vi "MotionMacro#CMDExecute.vi"(3 "ProgramRef":refnum<vi>, 4 "Command":string[](array[string]), 5 "ThreadsQueue":refnum<queue>[](array[refnum]), 6 "ThreadNo.":u32, 7 "ThreadModReceive":refnum<queue>[](array[refnum]), 8 "StackIn":cluster{"Program":i32, "Prog Index":i32}[](array[cluster]), 9 "ThreadInfoIn":T1) -> (0 "StackOut":cluster{"Program":i32, "Prog Index":i32}[](array[cluster]), 1 "ThreadInfoOut":T1, 2 "ErrorCode":string)   [LabVIEW 2020]
uses:
  MainFrame/Global.vi
panel:
  out "Macro":string[][](array[string])
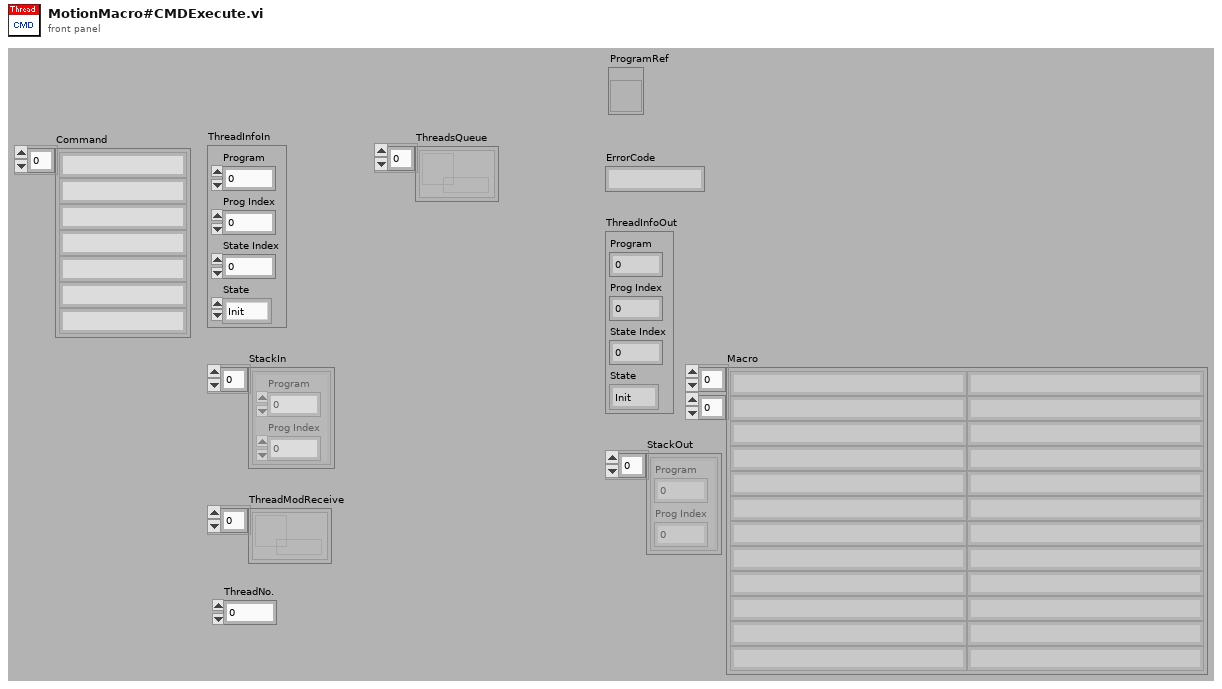
[diagram p1: front panel]
types:
  T1 = cluster{"Program":i32, "Prog Index":i32, "State Index":i32, "State":enum16{"Init", "Idle", "Auto Start", "Auto Running", "Step Start", "Step Running", "Suspend", "Restart", "Stop", "Reset"}}
  T2 = cluster{"指令":string, "代碼":string, "參數長度":i32, "乘數":dbl, "加數":dbl}[]
  T3 = enum16{"Get", "Init", "Set", "Delete", "GetElement", "Inc", "Dec", "ReName", "Copy"}
  T4 = enum16{"Init", "Idle", "Auto Start", "Auto Running", "Step Start", "Step Running", "Suspend", "Restart", "Stop", "Reset"}
  T5 = enum16{"Get", "UpdatePointS", "Init", "UpdateIndex", "GetCurrent&Index+1", "GetWithIndex", "ChkLast"}
  T6 = cluster{"指令":string, "代碼":string, "參數長度":i32, "乘數":dbl, "加數":dbl}[][]
  T7 = cluster{"指令":string, "代碼":string, "參數長度":i32, "乘數":dbl, "加數":dbl}
  T8 = cluster{cluster{"X":sgl, "Y":sgl, "Z":sgl, "U":sgl, "V":sgl, "W":sgl, "H":sgl}[]}
  T9 = cluster{"X":sgl, "Y":sgl, "Z":sgl, "U":sgl, "V":sgl, "W":sgl, "H":sgl}[]
  T10 = cluster{"X":sgl, "Y":sgl, "Z":sgl, "U":sgl, "V":sgl, "W":sgl, "H":sgl}
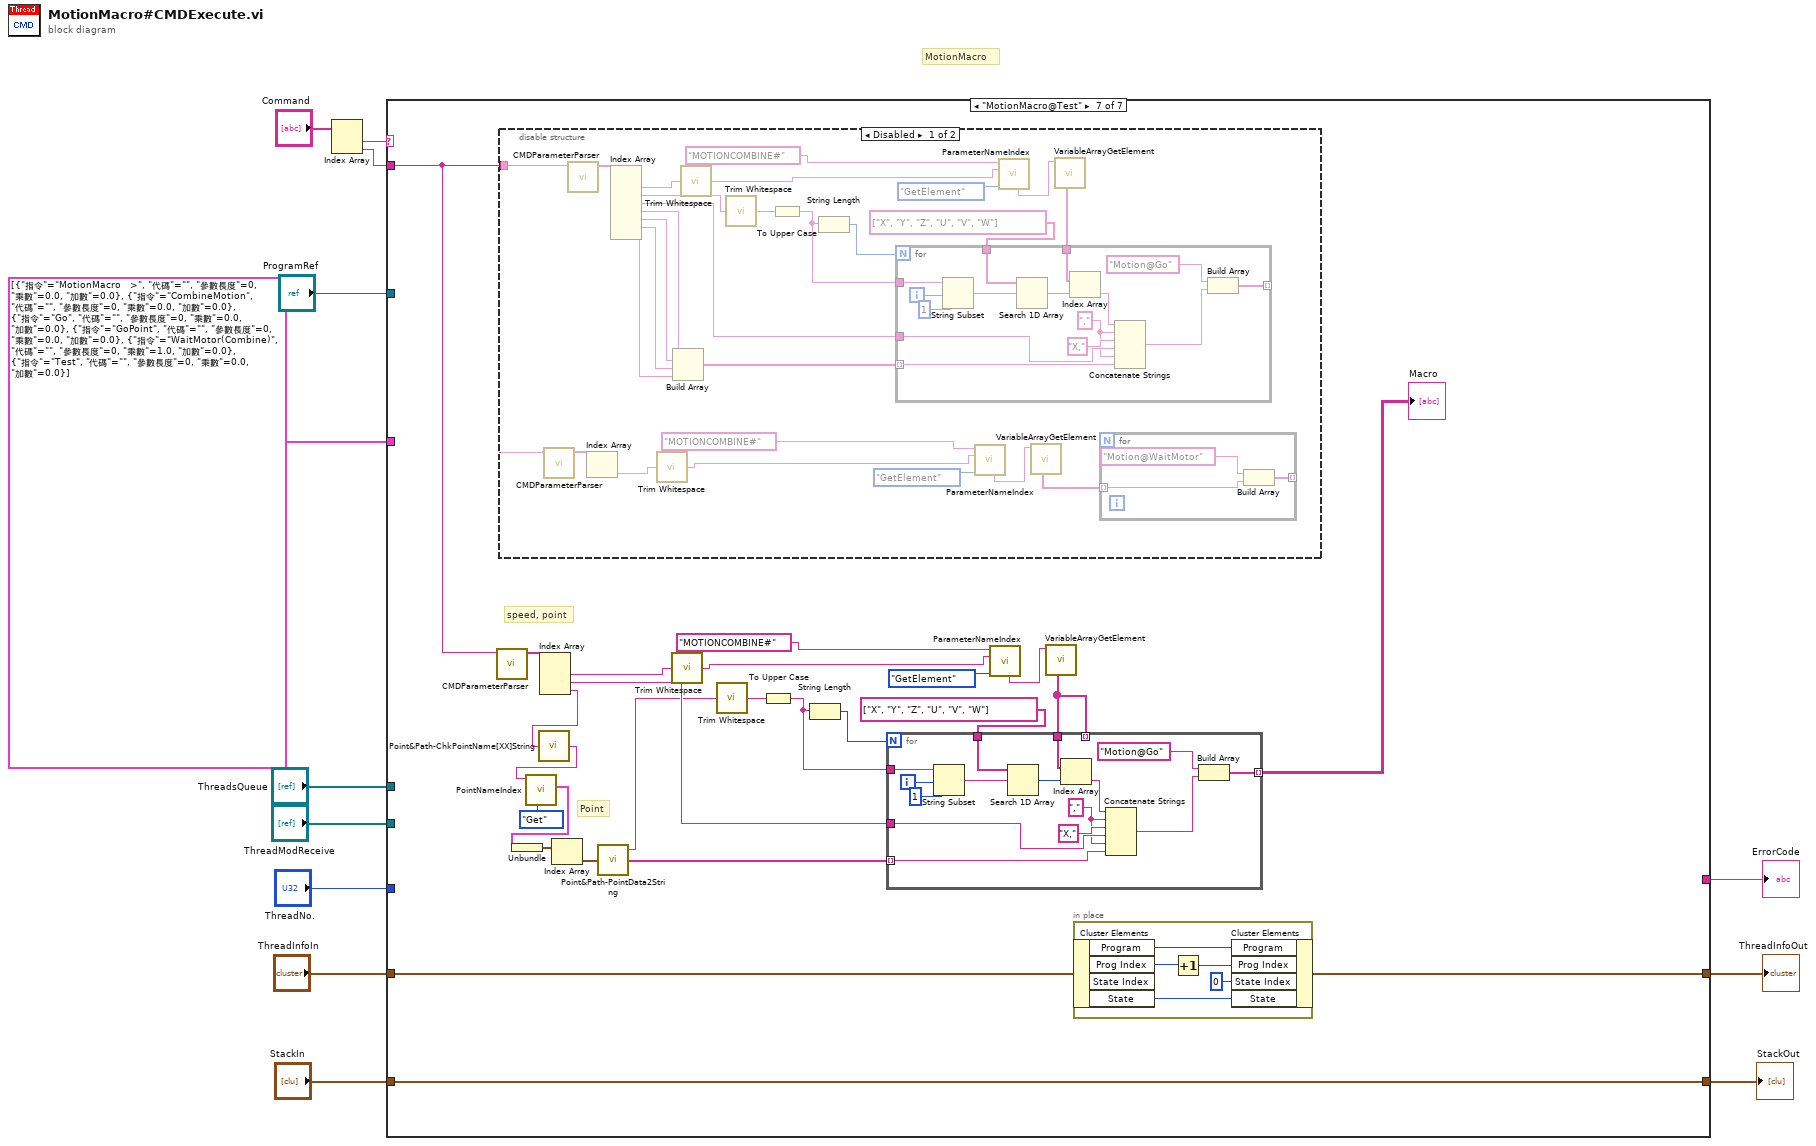
[diagram p0: block diagram]
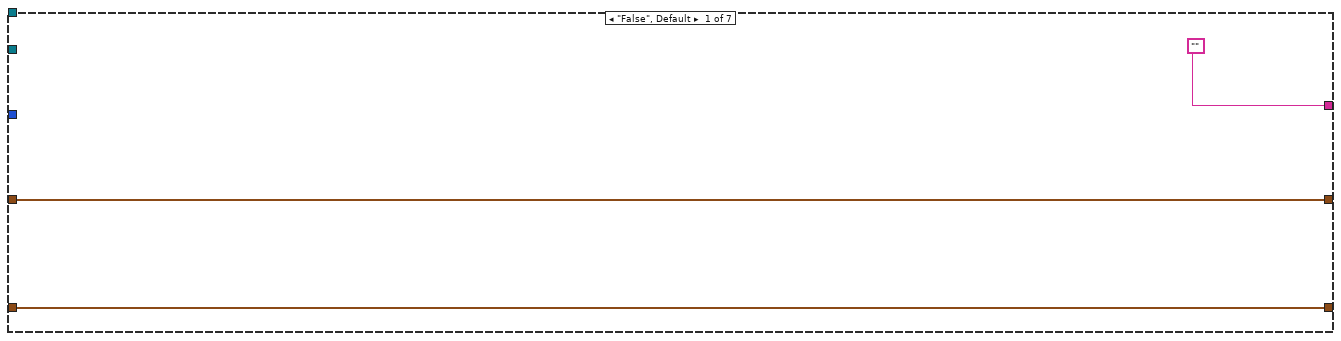
[diagram p2: hidden frame]
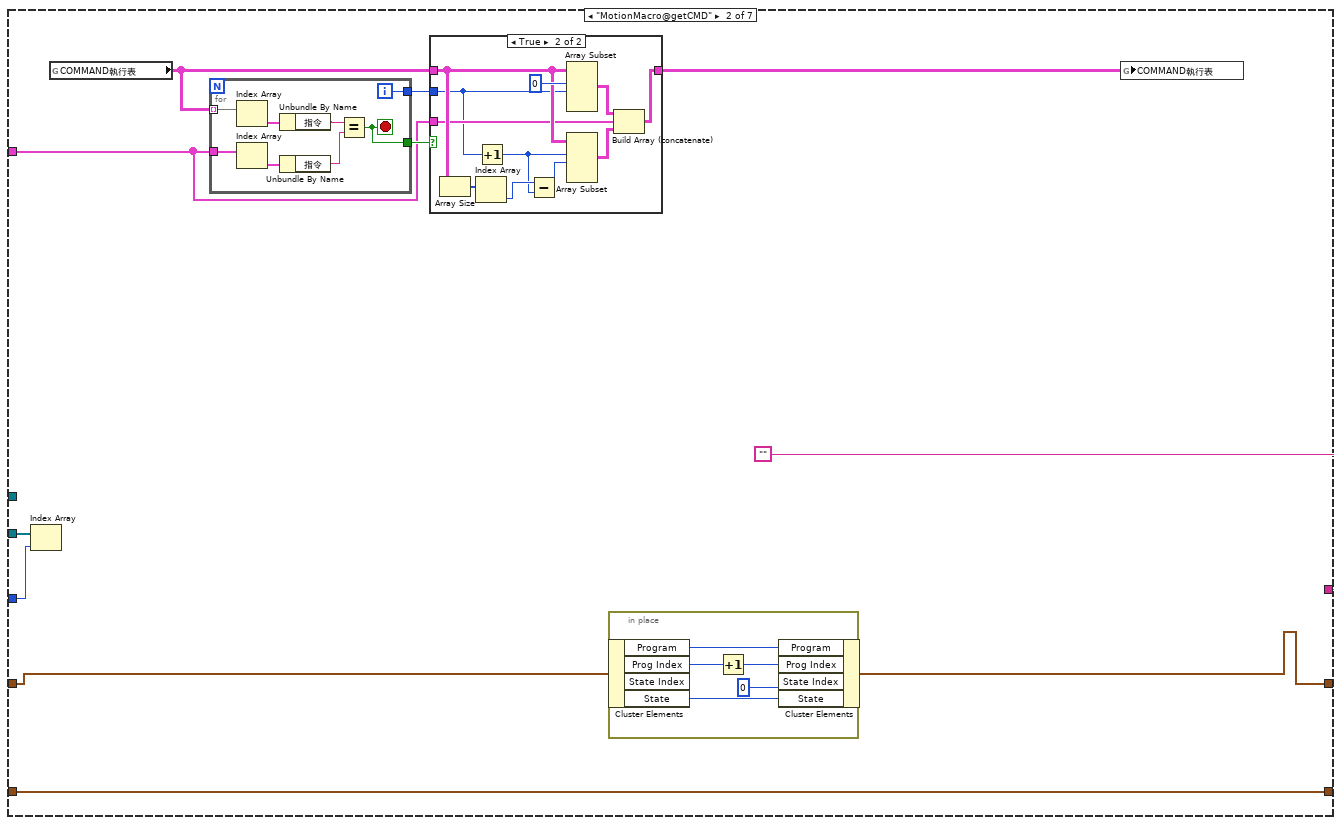
[diagram p3: hidden frame]
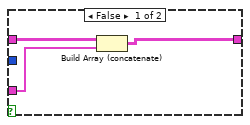
[diagram p4: hidden frame]
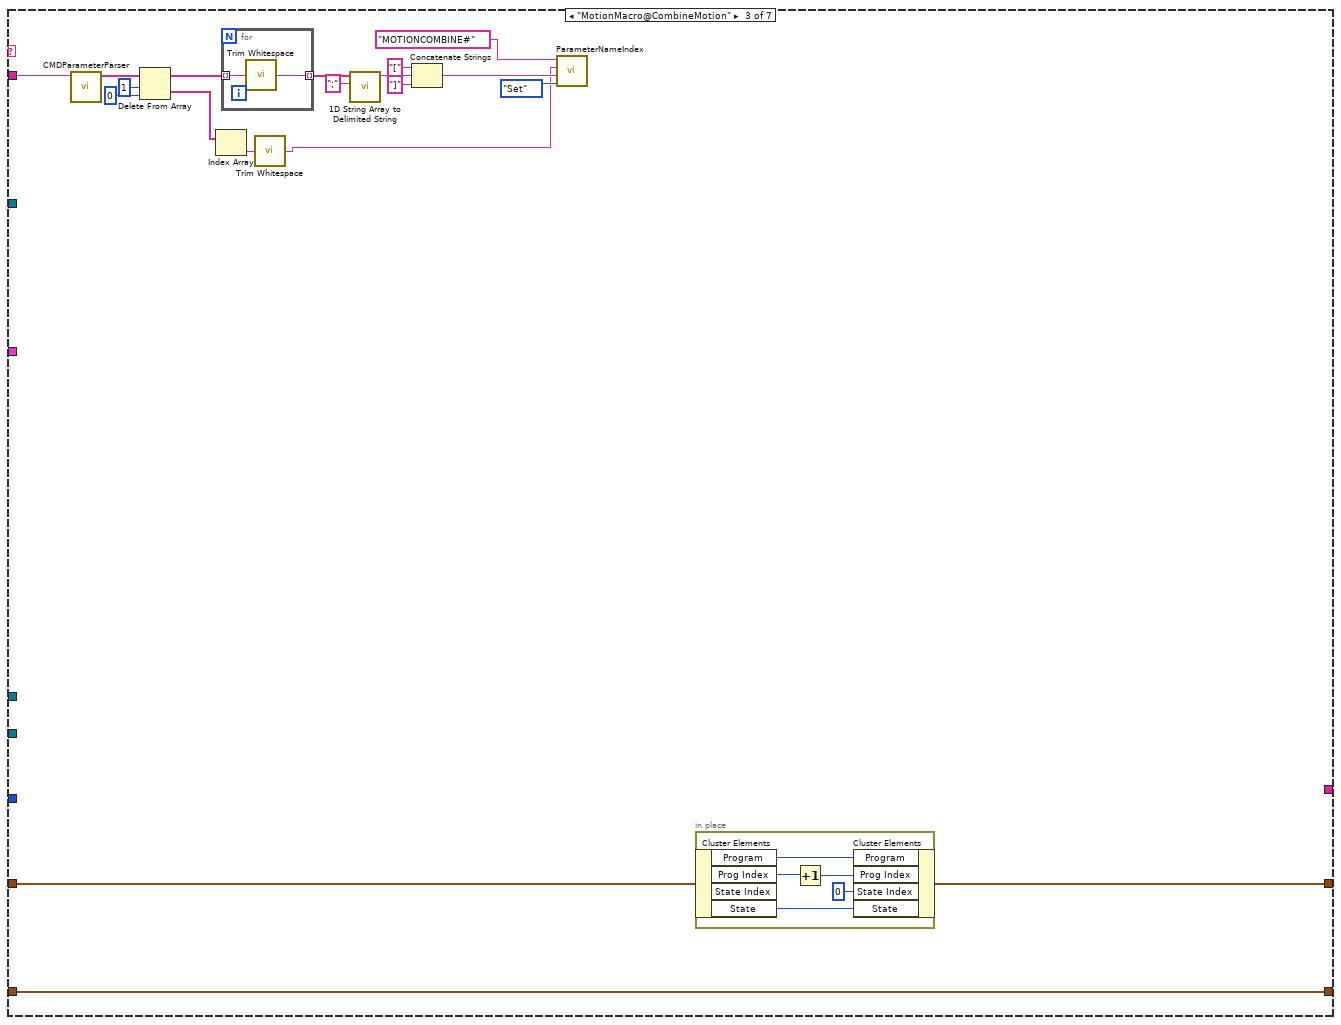
[diagram p5: hidden frame]
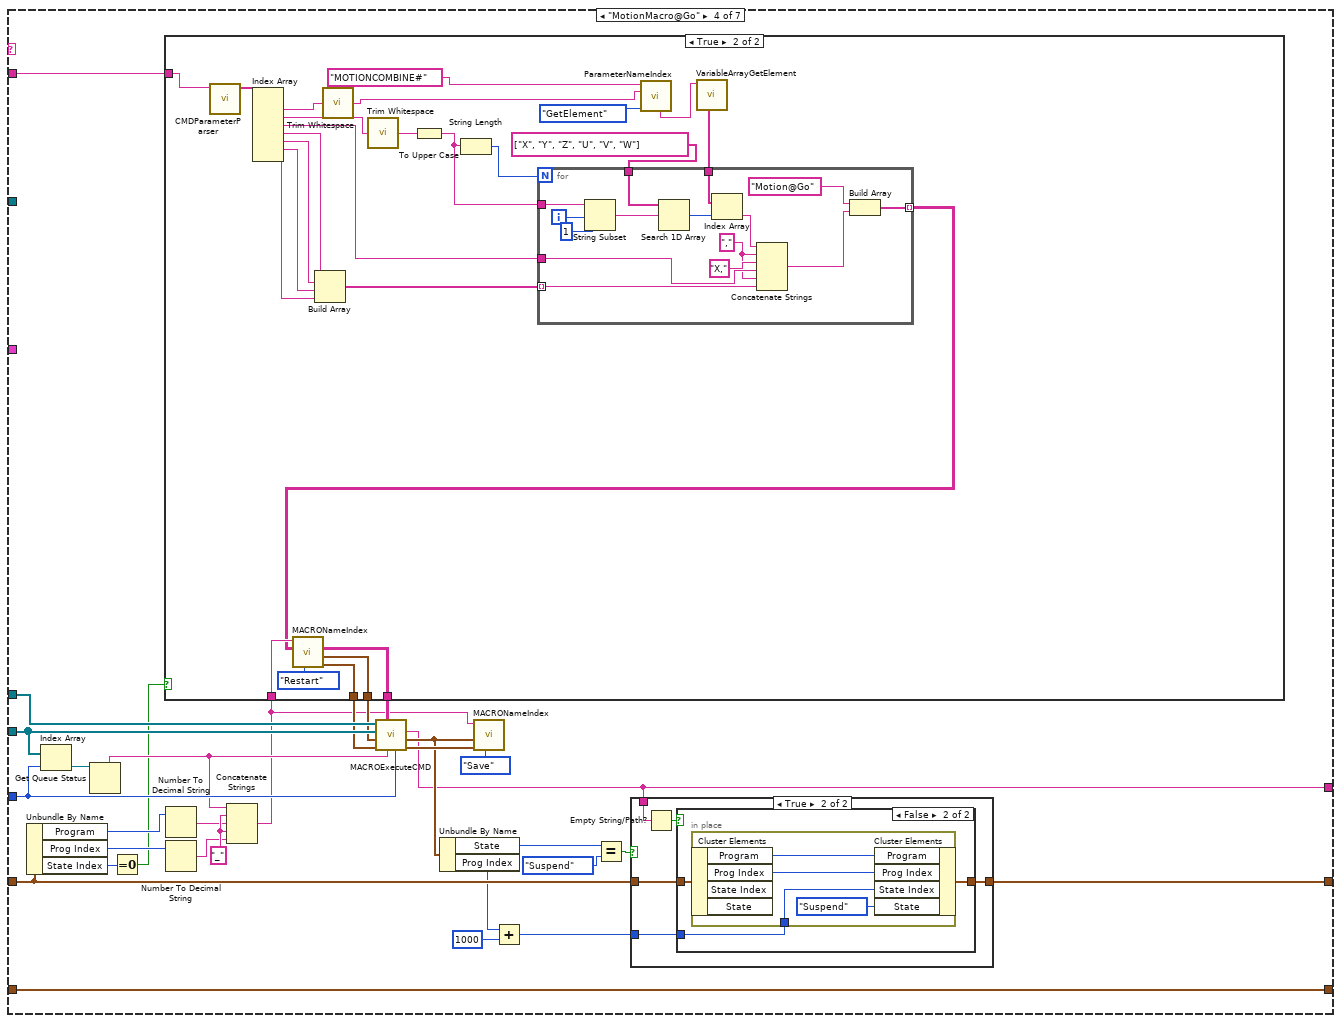
[diagram p6: hidden frame]
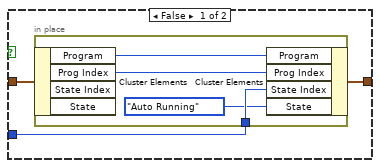
[diagram p7: hidden frame]
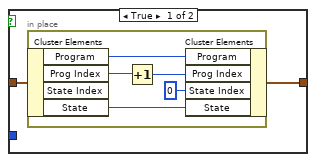
[diagram p8: hidden frame]
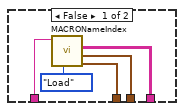
[diagram p9: hidden frame]
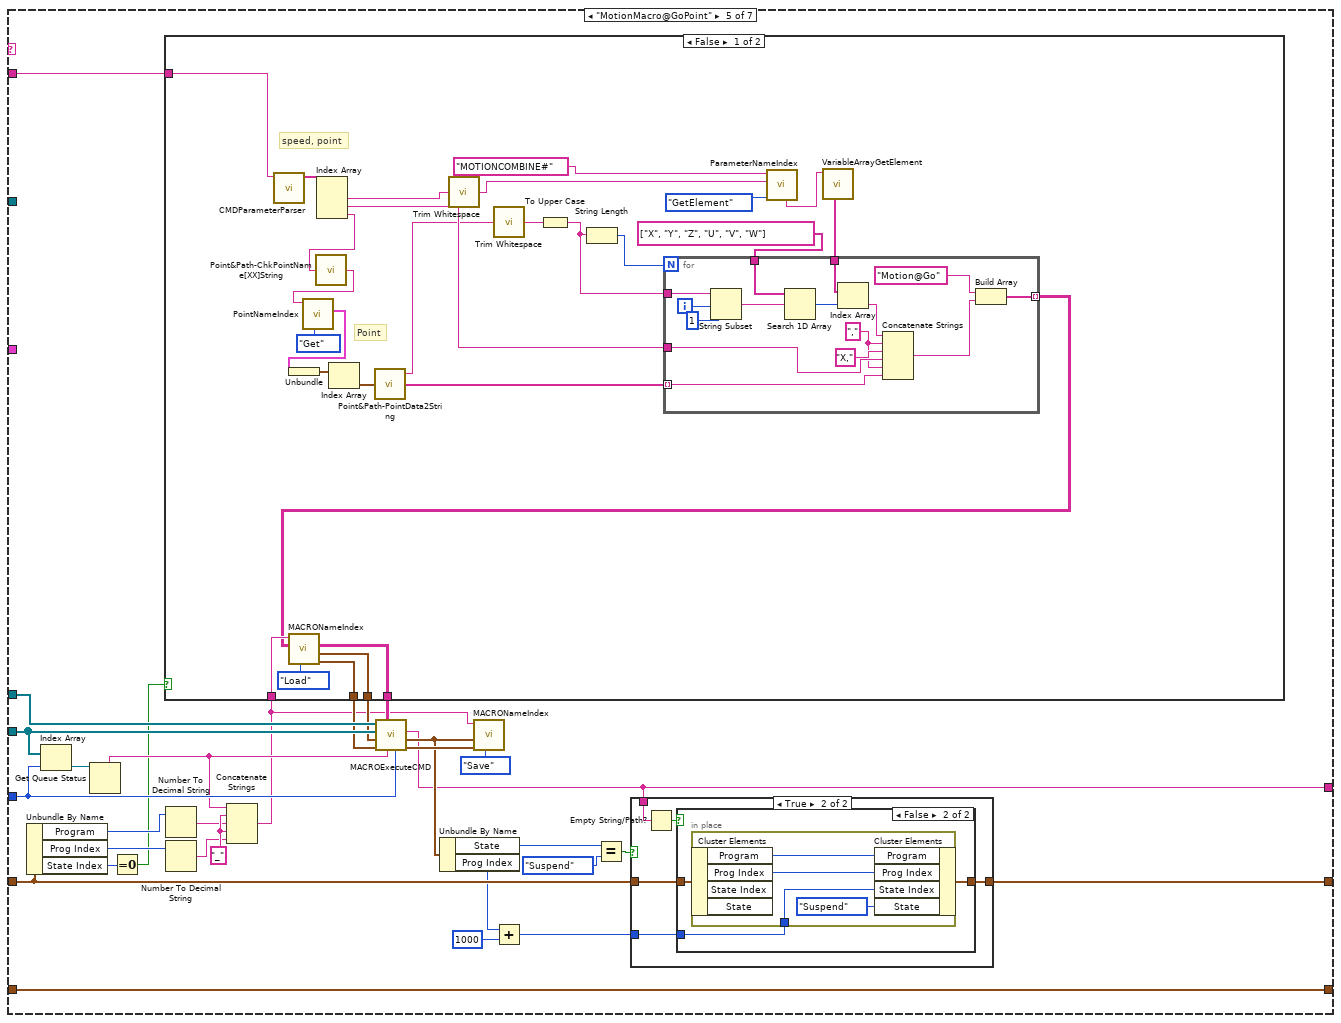
[diagram p10: hidden frame]
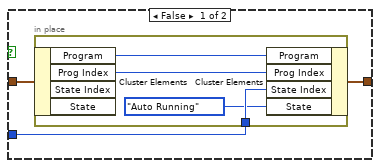
[diagram p11: hidden frame]
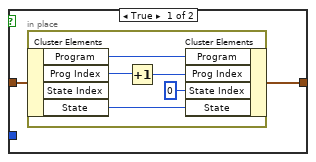
[diagram p12: hidden frame]
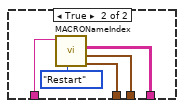
[diagram p13: hidden frame]
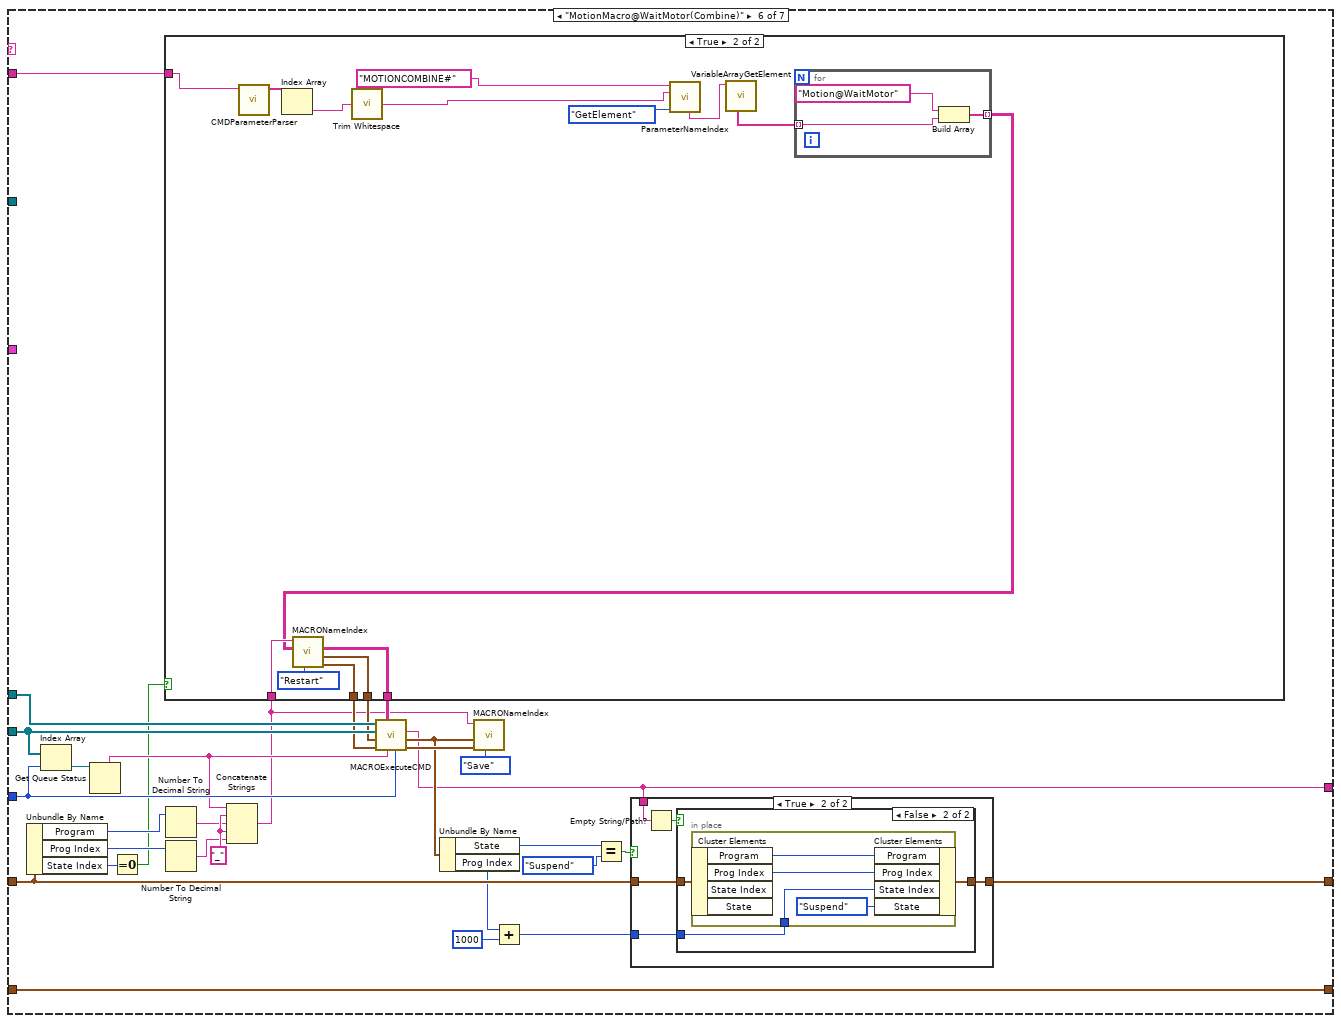
[diagram p14: hidden frame]
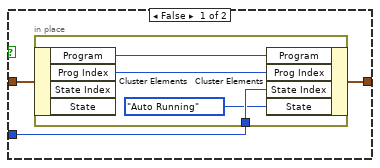
[diagram p15: hidden frame]
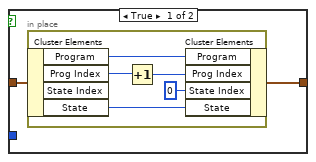
[diagram p16: hidden frame]
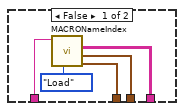
[diagram p17: hidden frame]
diagram:
  # "MotionMacro"
  n1 = Index Array(array="Command") -> (element #1=w1:string, element #2=w9:string)  [unwired: 2 in]
  n2 = case shown="\"MotionMacro@Test\"" w1 {
    tunnel: "ThreadModReceive" -> [_ w27 _ w92 w193 w296 _]
    tunnel: [w16 w25 w71 w94 w195 w298 w385] -> w6
    tunnel: "ThreadInfoIn" -> [w16 w24 w72 w95 w196 w299 w386]
    tunnel: "ThreadNo." -> [_ w26 _ w91 w192 w295 _]
    tunnel: w9 -> [_ _ w70 w109 w210 w313 w367]
    tunnel: "ThreadsQueue" -> [_ _ _ w93 w194 w297 _]
    tunnel: ["" "" _ w81 w182 w285 _] -> w11
    tunnel: [w14 w23 w73 w110 w211 w314 w387] -> w12
    tunnel: "StackIn" -> [w14 w23 w73 w110 w211 w314 w387]
    tunnel: T2 [{"指令"="MotionMacro   >", "代碼"="", "參數長度"=0, "乘數"=0.0, "加數"=0.0}, {"指令"="CombineMotion", "代碼"="", "參數長度"=0, "乘數"=0.0, "加數"=0.0}, {"指令"="Go", "代碼"="", "參數長度"=0, "乘數"=0.0, "加數"=0.0}, {"指令"="GoPoint", "代碼"="", "參數長度"=0, "乘數"=0.0, "加數"=0.0}, {"指令"="WaitMotor(Combine)", "代碼"="", "參數長度"=0, "乘數"=1.0, "加數"=0.0}, {"指令"="Test", "代碼"="", "參數長度"=0, "乘數"=0.0, "加數"=0.0}] ("Test程式表") -> [_ w19 _ _ _ _ _]
    tunnel: "ProgramRef" -> [_ _ _ _ _ _ _]
    frame "False", Default {
    }
    frame "MotionMacro@getCMD" {
      n3 = Index Array(array=w27, index=w26) -> ()  [unwired: 1 out]
      n4 = global read "Global.vi" "COMMAND執行表"() -> (w18:T6)
      n5 = for {
        tunnel: w18 -> [w47] mode=indexing
        tunnel: w19 -> [w48]
        tunnel: [w43] -> w20
        tunnel: [w42] -> w21
        i -> [w43]
        stop <- w42 stop-if-true
        n6 = Index Array(array=w47) -> (element=w49:T7)  [unwired: 1 in]
        n7 = Index Array(array=w48) -> (element=w46:T7)  [unwired: 1 in]
        n8 = Unbundle By Name(w49) -> ("指令"=w45:string)
        n9 = Unbundle By Name(w46) -> ("指令"=w44:string)
        n10 = Equal?(x=w45, y=w44) -> (x = y?=w42:bool)
      }
      n11 = case shown="True" w21 {
        tunnel: w20 -> [_ w32]
        tunnel: w19 -> [w29 w35]
        tunnel: w18 -> [w30 w40]
        tunnel: [w28 w33] -> w17
        frame False {
          n12 = Build Array (concatenate)(w30, w29) -> (w28:T6)
        }
        frame True {
          n13 = Array Size(array=w40) -> (size(s)=w39:i32[])
          n14 = Index Array(array=w39) -> (element=w38:i32)  [unwired: 1 in]
          n15 = Increment(x=w32) -> (x+1=w31:i32)
          n16 = Subtract(x=w38, y=w31) -> (x-y=w37:i32)
          n17 = Array Subset(array=w40, index (row)=0 ("index"), length (row)=w32) -> (w36:T6)  [unwired: 2 in]
          n18 = Array Subset(array=w40, index (row)=w31, length (row)=w37) -> (w34:T6)  [unwired: 2 in]
          n19 = Build Array (concatenate)(w36, w35, w34) -> (w33:T6)
        }
      }
      n20 = in-place {
        n21 = in-place-cluster #1(w24) -> ("Program"=w54:i32, "Prog Index"=w52:i32, "State"=w50:T4)  [unwired: 1 out]
        n22 = Increment(x=w52) -> (x+1=w53:i32)
        n23 = in-place-cluster #1("Program"=w54, "Prog Index"=w53, "State Index"=0, "State"=w50) -> (w25:T1)
      }
      n24 = global write "Global.vi" "COMMAND執行表"(w17) -> ()
    }
    frame "MotionMacro@CombineMotion" {
      n25 = call "CMDParameterParser.vi"("CMDParameter"=w70) -> ("Input"=w69:string[])  [unwired: 8 in, 2 out]
      n26 = Delete From Array(array=w69, length=1, index=0) -> (deleted portion=w62:string[], array with subset deleted=w58:string[])
      n27 = Index Array(array=w62) -> (element=w59:string)  [unwired: 1 in]
      n28 = for {
        tunnel: w58 -> [w75] mode=indexing
        tunnel: [w74] -> w57 mode=indexing
        n29 = call <vilib>:"Trim Whitespace.vi"("string"=w75) -> ("trimmed string"=w74:string)  [unwired: 1 in]
      }
      n30 = call <vilib>:"Trim Whitespace.vi"("string"=w59) -> ("trimmed string"=w55:string)  [unwired: 1 in]
      n31 = call <vilib>:"1D String Array to Delimited String.vi"("delimiter"=";", "string array"=w57) -> ("delimited string"=w65:string)  [unwired: 9 in]
      n32 = Concatenate Strings("[" ("string"), w65, "]" ("string")) -> (w61:string)
      n33 = call "ParameterNameIndex.vi"("OP"=T3."Set", "Value"=w61, "Key"=w55, "VariableSection"="MOTIONCOMBINE#" ("string")) -> ()  [unwired: 1 in, 7 out]
      n34 = in-place {
        n35 = in-place-cluster #2(w72) -> ("Program"=w80:i32, "Prog Index"=w79:i32, "State"=w76:T4)  [unwired: 1 out]
        n36 = Increment(x=w79) -> (x+1=w78:i32)
        n37 = in-place-cluster #2("Program"=w80, "Prog Index"=w78, "State Index"=0, "State"=w76) -> (w71:T1)
      }
    }
    frame "MotionMacro@Go" {
      w104 = "_" ("string")
      n38 = Unbundle By Name(w95) -> ("Program"=w106:i32, "Prog Index"=w105:i32, "State Index"=w107:i32)
      n39 = Index Array(array=w92, index=w91) -> (element=w108:refnum<queue>)
      n40 = Get Queue Status(queue=w108) -> (queue name=w90:string)  [unwired: 2 in, 7 out]
      n41 = Equal To 0?(x=w107) -> (x = 0?=w82:bool)
      n42 = Number To Decimal String(number=w106) -> (decimal integer string=w103:string)  [unwired: 1 in]
      n43 = Number To Decimal String(number=w105) -> (decimal integer string=w102:string)  [unwired: 1 in]
      n44 = Concatenate Strings(w90, w104, w103, w104, w102) -> (w86:string)
      n45 = case shown="True" w82 {
        tunnel: w109 -> [_ w145]
        tunnel: [w140 w164] -> w89
        tunnel: [w139 w165] -> w88
        tunnel: [w138 w163] -> w87
        tunnel: w86 -> [w137 w162]
        frame False {
          n46 = call "MACRONameIndex.vi"("OP"=enum16{"Init", "Restart", "Load", "Save"}."Load", "ID"=w137) -> ("StackOut"=w140:cluster{"Program":i32, "Prog Index":i32}[], "ThreadInfoOut"=w139:T1, "ProgramOut"=w138:string[][])  [unwired: 7 in]
        }
        frame True {
          n47 = call "CMDParameterParser.vi"("CMDParameter"=w145) -> ("Input"=w161:string[])  [unwired: 8 in, 2 out]
          n48 = Index Array(array=w161) -> (element #1=w159:string, element #2=w157:string, element #3=w152:string, element #4=w151:string, element #5=w150:string, element #6=w149:string, element #7=w148:string)  [unwired: 7 in]
          n49 = Build Array(w151, w150, w149, w148) -> (w147:string[])
          n50 = call <vilib>:"Trim Whitespace.vi"("string"=w159) -> ("trimmed string"=w142:string)  [unwired: 1 in]
          n51 = call <vilib>:"Trim Whitespace.vi"("string"=w157) -> ("trimmed string"=w156:string)  [unwired: 1 in]
          n52 = To Upper Case(1:w156) -> (0:w154:string)
          n53 = String Length(string=w154) -> (length=w155:i32)
          n54 = call "ParameterNameIndex.vi"("OP"=T3."GetElement", "Key"=w142, "VariableSection"="MOTIONCOMBINE#" ("string")) -> ("ElementValue"=w158:string)  [unwired: 2 in, 6 out]
          n55 = call "VariableArrayGetElement.vi"("String"=w158) -> ("Array"=w146:string[])  [unwired: 6 in, 4 out]
          n56 = for {
            N: w155 -> [_]
            tunnel: w146 -> [w176]
            tunnel: w154 -> [w181]
            tunnel: string[] ["X", "Y", "Z", "U", "V", "W"] -> [w178]
            tunnel: w152 -> [w171]
            tunnel: w147 -> [w169] mode=indexing
            tunnel: [w167] -> w144 mode=indexing
            i -> [w180]
            w170 = "," ("string")
            n57 = String Subset(string=w181, offset (0)=w180, length (rest)=1 ("length (rest)")) -> (substring=w177:string)
            n58 = Search 1D Array(1D array=w178, element=w177) -> (index of element=w175:i32)  [unwired: 1 in]
            n59 = Index Array(array=w176, index=w175) -> (element=w173:string)
            n60 = Concatenate Strings(w173, w170, "X," ("string"), w171, w170, w169) -> (w168:string)
            n61 = Build Array("Motion@Go" ("substring"), w168) -> (w167:string[])
          }
          n62 = call "MACRONameIndex.vi"("OP"=enum16{"Init", "Restart", "Load", "Save"}."Restart", "Program"=w144, "ID"=w162) -> ("StackOut"=w164:cluster{"Program":i32, "Prog Index":i32}[], "ThreadInfoOut"=w165:T1, "ProgramOut"=w163:string[][])  [unwired: 6 in]
        }
      }
      n63 = call "MACROExecuteCMD.vi"("ThreadNo"=w91, "ProgramSelect"=w90, "MacroProgram"=w87, "StackIn"=w89, "ThreadInfoIn"=w88, "Thread Mod ReciveS"=w92, "Threads"=w93) -> ("StackOut"=w100:cluster{"Program":i32, "Prog Index":i32}[], "ThreadInfoOut"=w99:T1, "ErrorOut"=w81:string)  [unwired: 2 in]
      n64 = Unbundle By Name(w99) -> ("State"=w98:T4, "Prog Index"=w84:i32)
      n65 = call "MACRONameIndex.vi"("OP"=enum16{"Init", "Restart", "Load", "Save"}."Save", "StackIn"=w100, "ThreadInfoIn"=w99, "ID"=w86) -> ()  [unwired: 5 in, 3 out]
      n66 = Add(x=w84, y=1000) -> (x+y=w85:i32)
      n67 = Equal?(x=w98, y=T4."Suspend") -> (x = y?=w96:bool)
      n68 = case shown="True" w96 {
        tunnel: w95 -> [w113 w122]
        tunnel: [w112 w121] -> w94
        tunnel: w85 -> [w111 w118]
        tunnel: w81 -> [_ w119]
        frame False {
          n69 = in-place {
            in-place-border: w111 -> [w115]
            n70 = in-place-cluster #3(w113) -> ("Program"=w117:i32, "Prog Index"=w116:i32)  [unwired: 2 out]
            n71 = in-place-cluster #3("Program"=w117, "Prog Index"=w116, "State Index"=w115, "State"=T4."Auto Running") -> (w112:T1)
          }
        }
        frame True {
          n72 = Empty String/Path?(string/path=w119) -> (empty?=w120:bool)
          n73 = case shown="False" w120 {
            tunnel: w122 -> [w124 w132]
            tunnel: [w123 w131] -> w121
            tunnel: w118 -> [_ w130]
            frame True {
              n74 = in-place {
                n75 = in-place-cluster #4(w124) -> ("Program"=w129:i32, "Prog Index"=w128:i32, "State"=w125:T4)  [unwired: 1 out]
                n76 = Increment(x=w128) -> (x+1=w127:i32)
                n77 = in-place-cluster #4("Program"=w129, "Prog Index"=w127, "State Index"=0, "State"=w125) -> (w123:T1)
              }
            }
            frame False {
              n78 = in-place {
                in-place-border: w130 -> [w133]
                n79 = in-place-cluster #5(w132) -> ("Program"=w136:i32, "Prog Index"=w135:i32)  [unwired: 2 out]
                n80 = in-place-cluster #5("Program"=w136, "Prog Index"=w135, "State Index"=w133, "State"=T4."Suspend") -> (w131:T1)
              }
            }
          }
        }
      }
    }
    frame "MotionMacro@GoPoint" {
      w205 = "_" ("string")
      n81 = Unbundle By Name(w196) -> ("Program"=w207:i32, "Prog Index"=w206:i32, "State Index"=w208:i32)
      n82 = Index Array(array=w193, index=w192) -> (element=w209:refnum<queue>)
      n83 = Get Queue Status(queue=w209) -> (queue name=w191:string)  [unwired: 2 in, 7 out]
      n84 = Equal To 0?(x=w208) -> (x = 0?=w183:bool)
      n85 = Number To Decimal String(number=w207) -> (decimal integer string=w204:string)  [unwired: 1 in]
      n86 = Number To Decimal String(number=w206) -> (decimal integer string=w203:string)  [unwired: 1 in]
      n87 = Concatenate Strings(w191, w205, w204, w205, w203) -> (w187:string)
      n88 = case shown="False" w183 {
        tunnel: w210 -> [w240 _]
        tunnel: [w263 w282] -> w190
        tunnel: [w262 w283] -> w189
        tunnel: [w261 w281] -> w188
        tunnel: w187 -> [w260 w280]
        frame False {
          # "speed, point"
          # "Point"
          n89 = call "CMDParameterParser.vi"("CMDParameter"=w240) -> ("Input"=w259:string[])  [unwired: 8 in, 2 out]
          n90 = Index Array(array=w259) -> (element #1=w257:string, element #2=w250:string, element #3=w244:string)  [unwired: 3 in]
          n91 = call "Point&Path-ChkPointName[XX]String.vi"("PointName[XX]"=w244) -> ("PointName"=w249:string)  [unwired: 2 in, 2 out]
          n92 = call "PointNameIndex.vi"("OP"=T5."Get", "PointName"=w249) -> ("PointDataOut"=w247:T8)  [unwired: 4 in, 5 out]
          n93 = Unbundle(w247) -> (w246:T9)
          n94 = Index Array(array=w246) -> (element=w245:T10)  [unwired: 1 in]
          n95 = call "Point&Path-PointData2String.vi"("Point"=w245) -> ("PositionStingArray"=w242:string[], "Axis"=w243:string)  [unwired: 2 in, 1 out]
          n96 = call <vilib>:"Trim Whitespace.vi"("string"=w257) -> ("trimmed string"=w238:string)  [unwired: 1 in]
          n97 = call <vilib>:"Trim Whitespace.vi"("string"=w243) -> ("trimmed string"=w255:string)  [unwired: 1 in]
          n98 = To Upper Case(1:w255) -> (0:w253:string)
          n99 = String Length(string=w253) -> (length=w254:i32)
          n100 = call "ParameterNameIndex.vi"("OP"=T3."GetElement", "Key"=w238, "VariableSection"="MOTIONCOMBINE#" ("string")) -> ("ElementValue"=w256:string)  [unwired: 2 in, 6 out]
          n101 = call "VariableArrayGetElement.vi"("String"=w256) -> ("Array"=w251:string[])  [unwired: 6 in, 4 out]
          n102 = for {
            N: w254 -> [_]
            tunnel: w251 -> [w274]
            tunnel: w253 -> [w279]
            tunnel: string[] ["X", "Y", "Z", "U", "V", "W"] -> [w276]
            tunnel: w250 -> [w269]
            tunnel: [w266] -> w241 mode=indexing
            tunnel: w242 -> [w265] mode=indexing
            i -> [w278]
            w268 = "," ("string")
            n103 = String Subset(string=w279, offset (0)=w278, length (rest)=1 ("length (rest)")) -> (substring=w275:string)
            n104 = Search 1D Array(1D array=w276, element=w275) -> (index of element=w273:i32)  [unwired: 1 in]
            n105 = Index Array(array=w274, index=w273) -> (element=w271:string)
            n106 = Concatenate Strings(w271, w268, "X," ("string"), w269, w268, w265) -> (w267:string)
            n107 = Build Array("Motion@Go" ("substring"), w267) -> (w266:string[])
          }
          n108 = call "MACRONameIndex.vi"("OP"=enum16{"Init", "Restart", "Load", "Save"}."Load", "Program"=w241, "ID"=w260) -> ("StackOut"=w263:cluster{"Program":i32, "Prog Index":i32}[], "ThreadInfoOut"=w262:T1, "ProgramOut"=w261:string[][])  [unwired: 6 in]
        }
        frame True {
          n109 = call "MACRONameIndex.vi"("OP"=enum16{"Init", "Restart", "Load", "Save"}."Restart", "ID"=w280) -> ("StackOut"=w282:cluster{"Program":i32, "Prog Index":i32}[], "ThreadInfoOut"=w283:T1, "ProgramOut"=w281:string[][])  [unwired: 7 in]
        }
      }
      n110 = call "MACROExecuteCMD.vi"("ThreadNo"=w192, "ProgramSelect"=w191, "MacroProgram"=w188, "StackIn"=w190, "ThreadInfoIn"=w189, "Thread Mod ReciveS"=w193, "Threads"=w194) -> ("StackOut"=w201:cluster{"Program":i32, "Prog Index":i32}[], "ThreadInfoOut"=w200:T1, "ErrorOut"=w182:string)  [unwired: 2 in]
      n111 = Unbundle By Name(w200) -> ("State"=w199:T4, "Prog Index"=w185:i32)
      n112 = call "MACRONameIndex.vi"("OP"=enum16{"Init", "Restart", "Load", "Save"}."Save", "StackIn"=w201, "ThreadInfoIn"=w200, "ID"=w187) -> ()  [unwired: 5 in, 3 out]
      n113 = Add(x=w185, y=1000) -> (x+y=w186:i32)
      n114 = Equal?(x=w199, y=T4."Suspend") -> (x = y?=w197:bool)
      n115 = case shown="True" w197 {
        tunnel: w196 -> [w214 w223]
        tunnel: [w213 w222] -> w195
        tunnel: w186 -> [w212 w219]
        tunnel: w182 -> [_ w220]
        frame False {
          n116 = in-place {
            in-place-border: w212 -> [w216]
            n117 = in-place-cluster #6(w214) -> ("Program"=w218:i32, "Prog Index"=w217:i32)  [unwired: 2 out]
            n118 = in-place-cluster #6("Program"=w218, "Prog Index"=w217, "State Index"=w216, "State"=T4."Auto Running") -> (w213:T1)
          }
        }
        frame True {
          n119 = Empty String/Path?(string/path=w220) -> (empty?=w221:bool)
          n120 = case shown="False" w221 {
            tunnel: w223 -> [w225 w233]
            tunnel: [w224 w232] -> w222
            tunnel: w219 -> [_ w231]
            frame True {
              n121 = in-place {
                n122 = in-place-cluster #7(w225) -> ("Program"=w230:i32, "Prog Index"=w229:i32, "State"=w226:T4)  [unwired: 1 out]
                n123 = Increment(x=w229) -> (x+1=w228:i32)
                n124 = in-place-cluster #7("Program"=w230, "Prog Index"=w228, "State Index"=0, "State"=w226) -> (w224:T1)
              }
            }
            frame False {
              n125 = in-place {
                in-place-border: w231 -> [w234]
                n126 = in-place-cluster #8(w233) -> ("Program"=w237:i32, "Prog Index"=w236:i32)  [unwired: 2 out]
                n127 = in-place-cluster #8("Program"=w237, "Prog Index"=w236, "State Index"=w234, "State"=T4."Suspend") -> (w232:T1)
              }
            }
          }
        }
      }
    }
    frame "MotionMacro@WaitMotor(Combine)" {
      w308 = "_" ("string")
      n128 = Unbundle By Name(w299) -> ("Program"=w310:i32, "Prog Index"=w309:i32, "State Index"=w311:i32)
      n129 = Index Array(array=w296, index=w295) -> (element=w312:refnum<queue>)
      n130 = Get Queue Status(queue=w312) -> (queue name=w294:string)  [unwired: 2 in, 7 out]
      n131 = Equal To 0?(x=w311) -> (x = 0?=w286:bool)
      n132 = Number To Decimal String(number=w310) -> (decimal integer string=w307:string)  [unwired: 1 in]
      n133 = Number To Decimal String(number=w309) -> (decimal integer string=w306:string)  [unwired: 1 in]
      n134 = Concatenate Strings(w294, w308, w307, w308, w306) -> (w290:string)
      n135 = case shown="True" w286 {
        tunnel: w313 -> [_ w349]
        tunnel: [w344 w357] -> w293
        tunnel: [w343 w358] -> w292
        tunnel: [w342 w356] -> w291
        tunnel: w290 -> [w341 w355]
        frame False {
          n136 = call "MACRONameIndex.vi"("OP"=enum16{"Init", "Restart", "Load", "Save"}."Load", "ID"=w341) -> ("StackOut"=w344:cluster{"Program":i32, "Prog Index":i32}[], "ThreadInfoOut"=w343:T1, "ProgramOut"=w342:string[][])  [unwired: 7 in]
        }
        frame True {
          n137 = call "CMDParameterParser.vi"("CMDParameter"=w349) -> ("Input"=w354:string[])  [unwired: 8 in, 2 out]
          n138 = Index Array(array=w354) -> (element=w352:string)  [unwired: 1 in]
          n139 = call <vilib>:"Trim Whitespace.vi"("string"=w352) -> ("trimmed string"=w346:string)  [unwired: 1 in]
          n140 = call "ParameterNameIndex.vi"("OP"=T3."GetElement", "Key"=w346, "VariableSection"="MOTIONCOMBINE#" ("string")) -> ("ElementValue"=w351:string)  [unwired: 2 in, 6 out]
          n141 = call "VariableArrayGetElement.vi"("String"=w351) -> ("Array"=w350:string[])  [unwired: 6 in, 4 out]
          n142 = for {
            tunnel: w350 -> [w361] mode=indexing
            tunnel: [w360] -> w348 mode=indexing
            n143 = Build Array("Motion@WaitMotor" ("substring"), w361) -> (w360:string[])
          }
          n144 = call "MACRONameIndex.vi"("OP"=enum16{"Init", "Restart", "Load", "Save"}."Restart", "Program"=w348, "ID"=w355) -> ("StackOut"=w357:cluster{"Program":i32, "Prog Index":i32}[], "ThreadInfoOut"=w358:T1, "ProgramOut"=w356:string[][])  [unwired: 6 in]
        }
      }
      n145 = call "MACROExecuteCMD.vi"("ThreadNo"=w295, "ProgramSelect"=w294, "MacroProgram"=w291, "StackIn"=w293, "ThreadInfoIn"=w292, "Thread Mod ReciveS"=w296, "Threads"=w297) -> ("StackOut"=w304:cluster{"Program":i32, "Prog Index":i32}[], "ThreadInfoOut"=w303:T1, "ErrorOut"=w285:string)  [unwired: 2 in]
      n146 = Unbundle By Name(w303) -> ("State"=w302:T4, "Prog Index"=w288:i32)
      n147 = call "MACRONameIndex.vi"("OP"=enum16{"Init", "Restart", "Load", "Save"}."Save", "StackIn"=w304, "ThreadInfoIn"=w303, "ID"=w290) -> ()  [unwired: 5 in, 3 out]
      n148 = Add(x=w288, y=1000) -> (x+y=w289:i32)
      n149 = Equal?(x=w302, y=T4."Suspend") -> (x = y?=w300:bool)
      n150 = case shown="True" w300 {
        tunnel: w299 -> [w317 w326]
        tunnel: [w316 w325] -> w298
        tunnel: w289 -> [w315 w322]
        tunnel: w285 -> [_ w323]
        frame False {
          n151 = in-place {
            in-place-border: w315 -> [w319]
            n152 = in-place-cluster #9(w317) -> ("Program"=w321:i32, "Prog Index"=w320:i32)  [unwired: 2 out]
            n153 = in-place-cluster #9("Program"=w321, "Prog Index"=w320, "State Index"=w319, "State"=T4."Auto Running") -> (w316:T1)
          }
        }
        frame True {
          n154 = Empty String/Path?(string/path=w323) -> (empty?=w324:bool)
          n155 = case shown="False" w324 {
            tunnel: w326 -> [w328 w336]
            tunnel: [w327 w335] -> w325
            tunnel: w322 -> [_ w334]
            frame True {
              n156 = in-place {
                n157 = in-place-cluster #10(w328) -> ("Program"=w333:i32, "Prog Index"=w332:i32, "State"=w329:T4)  [unwired: 1 out]
                n158 = Increment(x=w332) -> (x+1=w331:i32)
                n159 = in-place-cluster #10("Program"=w333, "Prog Index"=w331, "State Index"=0, "State"=w329) -> (w327:T1)
              }
            }
            frame False {
              n160 = in-place {
                in-place-border: w334 -> [w337]
                n161 = in-place-cluster #11(w336) -> ("Program"=w340:i32, "Prog Index"=w339:i32)  [unwired: 2 out]
                n162 = in-place-cluster #11("Program"=w340, "Prog Index"=w339, "State Index"=w337, "State"=T4."Suspend") -> (w335:T1)
              }
            }
          }
        }
      }
    }
    frame "MotionMacro@Test" {
      # "speed, point"
      # "Point"
      n163 = call "CMDParameterParser.vi"("CMDParameter"=w367) -> ("Input"=w384:string[])  [unwired: 8 in, 2 out]
      n164 = disable-structure shown="Disabled" {
        disable-tunnel: w367 -> [w392 _]
        frame Disabled {
          n165 = call "CMDParameterParser.vi"("CMDParameter"=w392) -> ("Input"=w397:string[])  [unwired: 8 in, 2 out]
          n166 = call "CMDParameterParser.vi"("CMDParameter"=w392) -> ("Input"=w413:string[])  [unwired: 8 in, 2 out]
          n167 = Index Array(array=w397) -> (element=w395:string)  [unwired: 1 in]
          n168 = Index Array(array=w413) -> (element #1=w411:string, element #2=w409:string, element #3=w404:string, element #4=w403:string, element #5=w402:string, element #6=w401:string, element #7=w400:string)  [unwired: 7 in]
          n169 = call <vilib>:"Trim Whitespace.vi"("string"=w395) -> ("trimmed string"=w388:string)  [unwired: 1 in]
          n170 = Build Array(w403, w402, w401, w400) -> (w399:string[])
          n171 = call <vilib>:"Trim Whitespace.vi"("string"=w411) -> ("trimmed string"=w391:string)  [unwired: 1 in]
          n172 = call <vilib>:"Trim Whitespace.vi"("string"=w409) -> ("trimmed string"=w408:string)  [unwired: 1 in]
          n173 = To Upper Case(1:w408) -> (0:w406:string)
          n174 = String Length(string=w406) -> (length=w407:i32)
          n175 = call "ParameterNameIndex.vi"("OP"=T3."GetElement", "Key"=w388, "VariableSection"="MOTIONCOMBINE#" ("string")) -> ("ElementValue"=w394:string)  [unwired: 2 in, 6 out]
          n176 = call "ParameterNameIndex.vi"("OP"=T3."GetElement", "Key"=w391, "VariableSection"="MOTIONCOMBINE#" ("string")) -> ("ElementValue"=w410:string)  [unwired: 2 in, 6 out]
          n177 = call "VariableArrayGetElement.vi"("String"=w394) -> ("Array"=w393:string[])  [unwired: 6 in, 4 out]
          n178 = call "VariableArrayGetElement.vi"("String"=w410) -> ("Array"=w398:string[])  [unwired: 6 in, 4 out]
          n179 = for {
            N: w407 -> [_]
            tunnel: w398 -> [w426]
            tunnel: w406 -> [w431]
            tunnel: string[] ["X", "Y", "Z", "U", "V", "W"] -> [w428]
            tunnel: w404 -> [w421]
            tunnel: w399 -> [w419] mode=indexing
            tunnel: [w417] -> _ mode=indexing
            i -> [w430]
            w420 = "," ("string")
            n180 = String Subset(string=w431, offset (0)=w430, length (rest)=1 ("length (rest)")) -> (substring=w427:string)
            n181 = Search 1D Array(1D array=w428, element=w427) -> (index of element=w425:i32)  [unwired: 1 in]
            n182 = Index Array(array=w426, index=w425) -> (element=w423:string)
            n183 = Concatenate Strings(w423, w420, "X," ("string"), w421, w420, w419) -> (w418:string)
            n184 = Build Array("Motion@Go" ("substring"), w418) -> (w417:string[])
          }
          n185 = for {
            tunnel: w393 -> [w415] mode=indexing
            tunnel: [w414] -> _ mode=indexing
            n186 = Build Array("Motion@WaitMotor" ("substring"), w415) -> (w414:string[])
          }
        }
        frame Enabled {
        }
      }
      n187 = Index Array(array=w384) -> (element #1=w382:string, element #2=w376:string, element #3=w370:string)  [unwired: 3 in]
      n188 = call "Point&Path-ChkPointName[XX]String.vi"("PointName[XX]"=w370) -> ("PointName"=w375:string)  [unwired: 2 in, 2 out]
      n189 = call "PointNameIndex.vi"("OP"=T5."Get", "PointName"=w375) -> ("PointDataOut"=w373:T8)  [unwired: 4 in, 5 out]
      n190 = Unbundle(w373) -> (w372:T9)
      n191 = Index Array(array=w372) -> (element=w371:T10)  [unwired: 1 in]
      n192 = call "Point&Path-PointData2String.vi"("Point"=w371) -> ("PositionStingArray"=w368:string[], "Axis"=w369:string)  [unwired: 2 in, 1 out]
      n193 = call <vilib>:"Trim Whitespace.vi"("string"=w382) -> ("trimmed string"=w363:string)  [unwired: 1 in]
      n194 = call <vilib>:"Trim Whitespace.vi"("string"=w369) -> ("trimmed string"=w380:string)  [unwired: 1 in]
      n195 = To Upper Case(1:w380) -> (0:w378:string)
      n196 = String Length(string=w378) -> (length=w379:i32)
      n197 = call "ParameterNameIndex.vi"("OP"=T3."GetElement", "Key"=w363, "VariableSection"="MOTIONCOMBINE#" ("string")) -> ("ElementValue"=w381:string)  [unwired: 2 in, 6 out]
      n198 = call "VariableArrayGetElement.vi"("String"=w381) -> ("Array"=w365:string[])  [unwired: 6 in, 4 out]
      n199 = for {
        N: w379 -> [_]
        tunnel: w365 -> [w441]
        tunnel: w378 -> [w446]
        tunnel: string[] ["X", "Y", "Z", "U", "V", "W"] -> [w443]
        tunnel: w376 -> [w436]
        tunnel: [w433] -> w366 mode=indexing
        tunnel: w368 -> [w432] mode=indexing
        tunnel: w365 -> [_] mode=indexing
        i -> [w445]
        w435 = "," ("string")
        n200 = String Subset(string=w446, offset (0)=w445, length (rest)=1 ("length (rest)")) -> (substring=w442:string)
        n201 = Search 1D Array(1D array=w443, element=w442) -> (index of element=w440:i32)  [unwired: 1 in]
        n202 = Index Array(array=w441, index=w440) -> (element=w438:string)
        n203 = Concatenate Strings(w438, w435, "X," ("string"), w436, w435, w432) -> (w434:string)
        n204 = Build Array("Motion@Go" ("substring"), w434) -> (w433:string[])
      }
      "Macro" <- w366
      n205 = in-place {
        n206 = in-place-cluster #12(w386) -> ("Program"=w451:i32, "Prog Index"=w450:i32, "State"=w447:T4)  [unwired: 1 out]
        n207 = Increment(x=w450) -> (x+1=w449:i32)
        n208 = in-place-cluster #12("Program"=w451, "Prog Index"=w449, "State Index"=0, "State"=w447) -> (w385:T1)
      }
    }
  }
  "StackOut" <- w12
  "ErrorCode" <- w11
  "ThreadInfoOut" <- w6
